vi "Check DC_2.vi"(0 "NXT":T3, 2 "DC Motors":T2={"DC Motor"=enum."DC Motor", "Address"=-1, "Address"=-1}) -> (4 "NXT":T3, 6 "Position 1":i32, 8 "Moving 1":bool, 10 "Position 2":i32, 15 "Moving 2":bool)   [LabVIEW 2012, in "4134Outputs.lvlib"]
uses:
  4134Outputs.lvlib
  <vilib>/NXT/Subs/LVHSConnector.ctl
  <vilib>/NXT/LegoClasses/BrickReference/BrickReference.lvclass
  <vilib>/NXT/Subs/MotorXNode.DC Motor Type.ctl
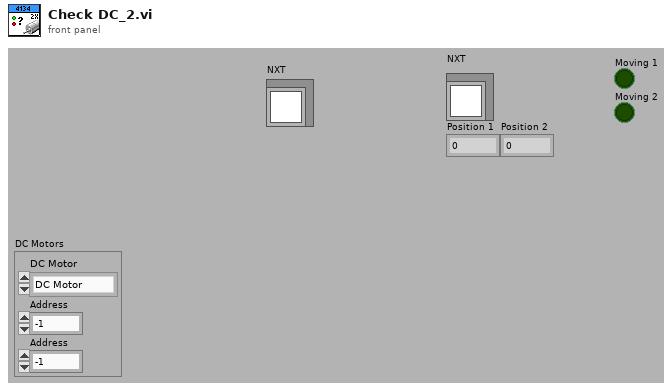
[diagram p1: front panel]
types:
  T1 = typedef "MotorXNode.DC Motor Type.ctl" = enum16{"DC Motor"}
  T2 = cluster{"DC Motor":T1, "Address":i16, "Address":i16}
  T3 = typedef "LVHSConnector.ctl" = refnum<class "BrickReference.lvclass">
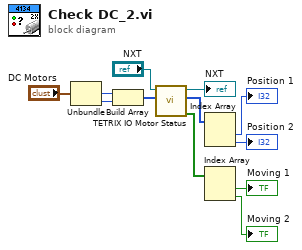
[diagram p0: block diagram]
diagram:
  n1 = Unbundle("DC Motors") -> ("Address"=w12:i16, "Address"=w10:i16)  [unwired: 1 out]
  n2 = Build Array(w12, w10) -> (w9:i16[])
  n3 = call <vilib>:"TETRIX IO Motor Status.vi"("DC Motors"=w9, "NXT"="NXT") -> ("Moves in Progress?"=w5:bool[], "Absolute Motor Positions"=w6:i32[], "NXT"=→"NXT":T3)  [unwired: 7 in]
  n4 = Index Array(array=w6) -> (element #1=→"Position 1":i32, element #2=→"Position 2":i32)  [unwired: 2 in]
  n5 = Index Array(array=w5) -> (element #1=→"Moving 1":bool, element #2=→"Moving 2":bool)  [unwired: 2 in]
